vi "QT_DynCall.vi"(0 "QT Ref In":T11, 1 "Frame Grabber Settings":T15={"Name"="", "Digitizer"=0, "Input"=0, "Width"=0, "Height"=0, "Input format"=enum."PAL", "Frame rate"=0.0, "Reserved"=0, "Dialogs"=0} {"Frame rate" format="%#1_6g"; "Dialogs" format="%.0b"}, 3 "Compression Settings":T14 {"Dialogs" format="%.0b"; "Comp. Quality" format="%.0x"; "Codec" format="%.0x"}, 4 "Movie Settings":T10 {"Dialogs" format="%.0b"}, 5 "Image in":T5 {"Dialogs" format="%.0b"}, 6 "Sound in":T4 {"Rate" format="%x"}, 7 "error in (no error)":errorcluster, 8 "Selector":T16=enum."Get QT & CIN info", 9 "Video Settings in":T3={"Color format"=1, "Hue"=0.0, "Saturation"=0.0, "Brightness"=0.0, "Contrast"=0.0, "Sharpness"=0.0, "Black Level"=0.0, "White Level"=0.0, "Options"=0, "Dialogs"=0} {"Dialogs" format="%.0b"; "Color format" items=["Black & White (8 bits)", "RGB (24 bits)", "RGBx (32 bits)", "RGBA (32bits)", "RGB B&W (32 bits)", "HSI (24 bits)", "HSIx (32 bits)", "HSI B&W (32 bits)"]; "Brightness" format="%.2f"; "Contrast" format="%.2f"; "Sharpness" format="%.2f"; "Black Level" format="%.2f"; "White Level" format="%.2f"; "Saturation" format="%.2f"; "Hue" format="%.2f"}, 12 "Private":T6={"reserved 1"=4, "reserved 2"=0, "reserved 3"=0, "reserved 4"=0}, 13 "Effect":T9 {"Matrix" format="%.2f"}, 15 "File Settings":T13 {"Dialogs" format="%.0b"}) -> (16 "Info Out":T12, 17 "Video Settings out":T3={"Color format"=1, "Hue"=0.0, "Saturation"=0.0, "Brightness"=0.0, "Contrast"=0.0, "Sharpness"=0.0, "Black Level"=0.0, "White Level"=0.0, "Options"=0, "Dialogs"=0} {"Dialogs" format="%.0b"; "Color format" items=["Black & White (8 bits)", "RGB (24 bits)", "RGBx (32 bits)", "RGBA (32bits)", "RGB B&W (32 bits)", "HSI (24 bits)", "HSIx (32 bits)", "HSI B&W (32 bits)"]; "Brightness" format="%.2f"; "Contrast" format="%.2f"; "Sharpness" format="%.2f"; "Black Level" format="%.2f"; "White Level" format="%.2f"; "Saturation" format="%.2f"; "Hue" format="%.2f"}, 20 "QT Ref Out":T11, 23 "Movie info":T7 {"Tracks"."Rate" format="%.2f"}, 24 "QT Info":T1 {"Digitizers"."In Flags" format="%.0b"; "Digitizers"."Out Flags" format="%.0b"; "Digitizers"."Inputs" items=["Composite", "S-Video", "RGB", "RGB Synch", "YUV", "YUV Synch", "TV Tuner", "sdiln"]; "CIN rev ID" format="%.2f"}, 25 "Image/Movie Out":T5 {"Dialogs" format="%.0b"}, 26 "Sound out":T4 {"Rate" format="%x"}, 27 "error out":errorcluster={"status"=TRUE, "code"=-43, "source"=""})   [LabVIEW 2024]
uses:
  <userlib>/ImageProcessing/QTLIB_2595_LV86/QT_Image.ctl
  <userlib>/ImageProcessing/QTLIB_2595_LV86/QT_Digitizer.ctl
  <userlib>/ImageProcessing/QTLIB_2595_LV86/QT_Info.ctl
  <userlib>/ImageProcessing/QTLIB_2595_LV86/QT_Selector.ctl
  <userlib>/ImageProcessing/QTLIB_2595_LV86/QT_Ref.ctl
  <userlib>/ImageProcessing/QTLIB_2595_LV86/QT_Sound.ctl
  <userlib>/ImageProcessing/QTLIB_2595_LV86/QT_Video.ctl
  <userlib>/ImageProcessing/QTLIB_2595_LV86/QT_ErrInfo.ctl
  <userlib>/ImageProcessing/QTLIB_2595_LV86/QT_Private.ctl
  <userlib>/ImageProcessing/QTLIB_2595_LV86/QT_Compression.ctl
  <userlib>/ImageProcessing/QTLIB_2595_LV86/QT_File.ctl
  <userlib>/ImageProcessing/QTLIB_2595_LV86/QT_FrameGrabber.ctl
  <userlib>/ImageProcessing/QTLIB_2595_LV86/QT_Track.ctl
  <userlib>/ImageProcessing/QTLIB_2595_LV86/QT_MovieInfo.ctl
  <userlib>/ImageProcessing/QTLIB_2595_LV86/QT_Movie.ctl
  <userlib>/ImageProcessing/QTLIB_2595_LV86/QT_Effect.ctl
panel:
  # "[0,0] [0,1]  [0,2] [1,0].. [2,2]"
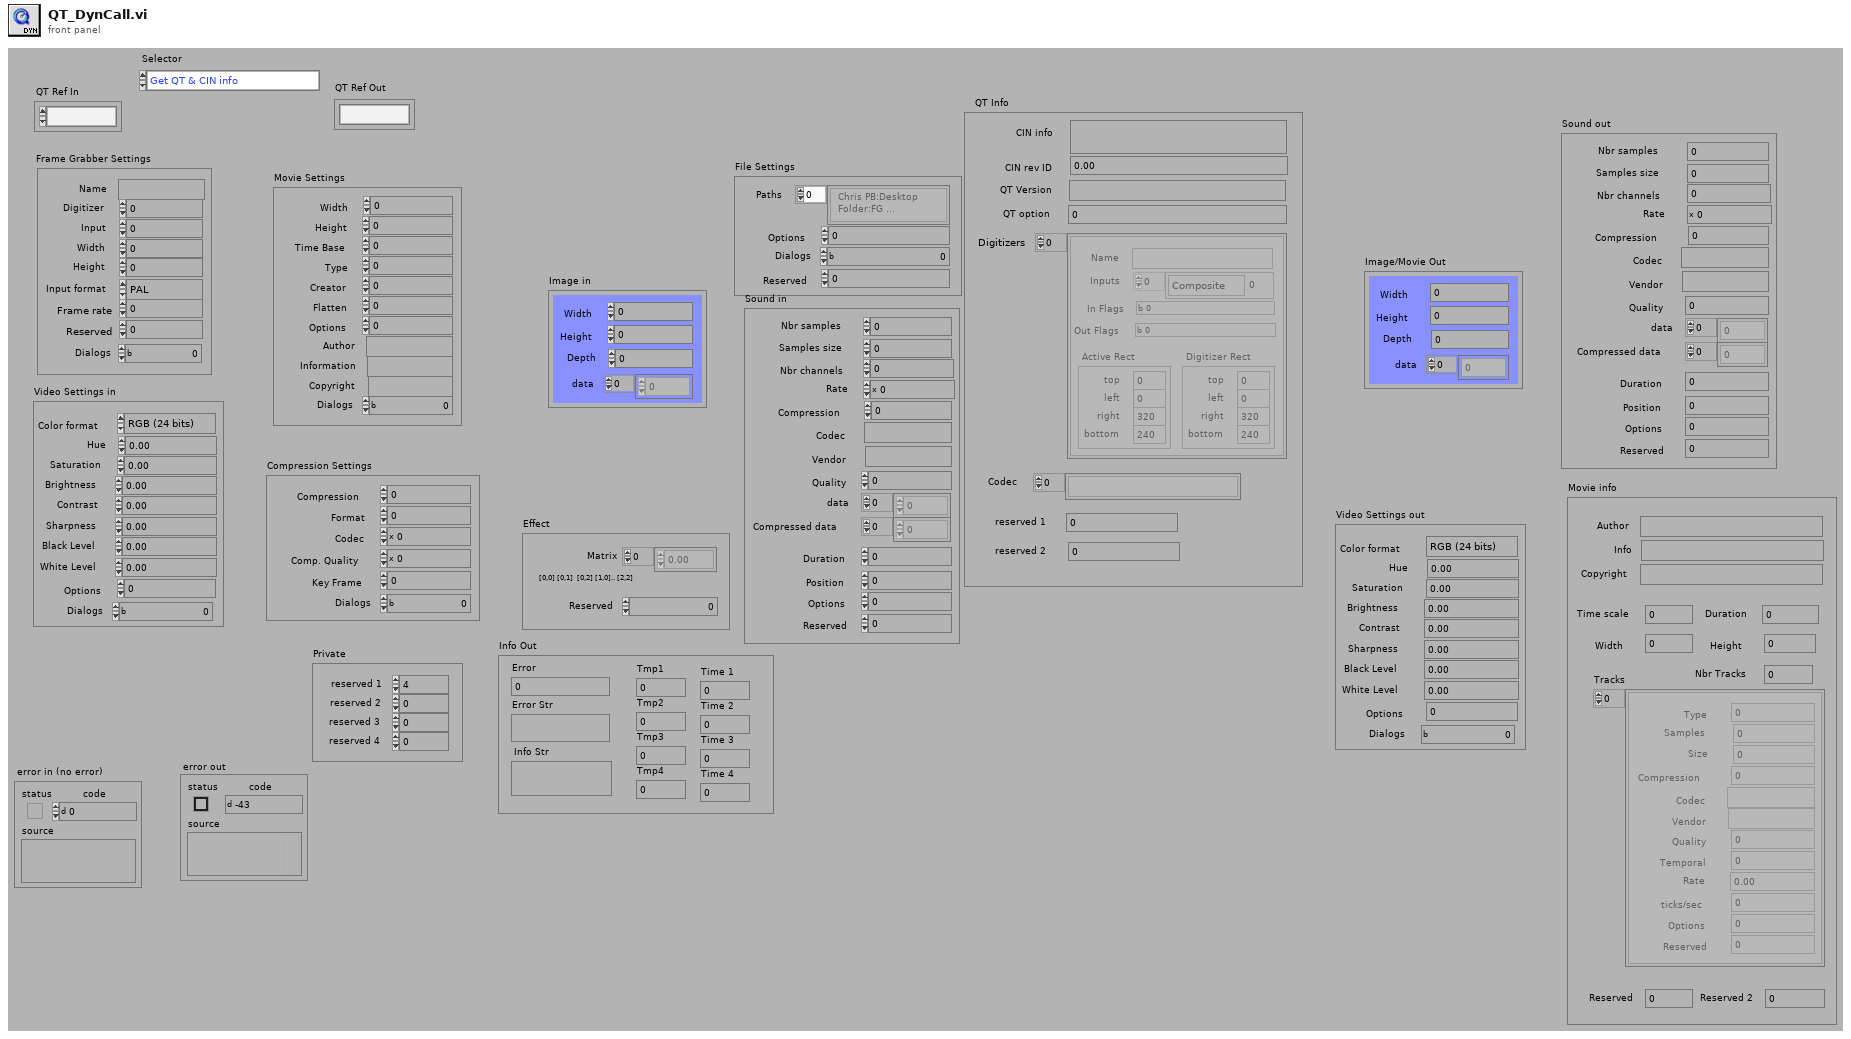
[diagram p1: front panel]
types:
  T1 = typedef "QT_Info.ctl" = cluster{"CIN info":string, "CIN rev ID":dbl, "QT Version":string, "QT option":i32, "Digitizers\n":T2[], "Codec":string[], "reserved 1":i32, "reserved 2":i32}
  T2 = typedef "QT_Digitizer.ctl" = cluster{"Name":string, "Inputs":i32[], "In Flags":i32, "Out Flags":i32, "Digitizer Rect":cluster{"top":i32, "left":i32, "right":i32, "bottom":i32}, "Active Rect":cluster{"top":i32, "left":i32, "right":i32, "bottom":i32}}
  T3 = typedef "QT_Video.ctl" = cluster{"Color format":u32, "Hue":dbl, "Saturation":dbl, "Brightness":dbl, "Contrast":dbl, "Sharpness":dbl, "Black Level":dbl, "White Level":dbl, "Options":i32, "Dialogs":u32}
  T4 = typedef "QT_Sound.ctl" = cluster{"Nbr samples":i32, "Samples size":i32, "Nbr channels":i32, "Rate ":i32, "Compression":i32, "Codec":string, "Vendor":string, "Quality":i32, "data":i16[], "Compressed data":u8[], "Duration":i32, "Position":i32, "Options":i32, "Reserved":i32}
  T5 = typedef "QT_Image.ctl" = cluster{"Width":i32, "Height":i32, "Depth":i32, "data":u8[], "Compressed data":u8[], "Color table":u32[], "Duration":i32, "Options":i32, "Timestamp":i32, "ID":i32, "Reserved":i32, "Dialogs":u32}
  T6 = typedef "QT_Private.ctl" = cluster{"reserved 1":i32, "reserved 2":i32, "reserved 3":i32, "reserved 4":i32}
  T7 = typedef "QT_MovieInfo.ctl" = cluster{"Author":string, "Info":string, "Copyright":string, "Time scale":i32, "Duration":i32, "Width":i32, "Height":i32, "Nbr Tracks":i32, "Tracks":T8[], "Reserved":i32, "Reserved 2":i32}
  T8 = typedef "QT_Track.ctl" = cluster{"Type":i32, "Samples":i32, "Size":i32, "Compression":i32, "Codec":string, "Vendor":string, "Quality":i32, "Temporal":i32, "Rate ":dbl, "ticks/sec":i32, "Options":i32, "Reserved":i32}
  T9 = typedef "QT_Effect.ctl" = cluster{"Reserved":i32, "Matrix":dbl[]}
  T10 = typedef "QT_Movie.ctl" = cluster{"Width":i32, "Height":i32, "Time Base":i32, "Type":i32, "Creator":i32, "Flatten":i32, "Options":i32, "Author":string, "Information":string, "Copyright":string, "Dialogs":u32}
  T11 = typedef "QT_Ref.ctl" = refnum<k1>
  T12 = typedef "QT_ErrInfo.ctl" = cluster{"Error":i32, "Error Str":string, "Info Str":string, "Tmp1":i32, "Tmp2":i32, "Tmp3":i32, "Tmp4":i32, "Time 1":i32, "Time 2":i32, "Time 3":i32, "Time 4":i32}
  T13 = typedef "QT_File.ctl" = cluster{"Paths":string[], "Options":i32, "Dialogs":u32, "Reserved":i32}
  T14 = typedef "QT_Compression.ctl" = cluster{"Compression":i32, "Format":i32, "Codec":i32, "Comp. Quality":i32, "Key Frame":i32, "Dialogs":u32}
  T15 = typedef "QT_FrameGrabber.ctl" = cluster{"Name":string, "Digitizer":i32, "Input":i32, "Width":i32, "Height":i32, "Input format":enum32{"NTSC", "PAL", "Secam"}, "Frame rate":dbl, "Reserved":i32, "Dialogs":u32}
  T16 = typedef "QT_Selector.ctl" = enum32{"do nothing", "Get all Sources", "Get Source info", "Open Image", "Save Image to File", "Effect", "Close", "SG Grab", "Compress in Memory", "Decompress to Memory", "New Movie", "Open Movie", "Add Frame", "Get Frame", "Close Movie", "Get QT & CIN info", "SG init", "SG Close", "Open sound file", "Close sound file", "Read sound data", "Write sound data", "Import sound", "Export sound", "Add sound to movie", "Get sound from movie", "reserved", "reserved 1", "reserved 2"}
  T17 = enum32{"invalid CPU target", "Motorola 68K", "PowerPC", "Intel x86", "SPARC", "PA-RISC", "MIPS", "Alpha"}
  T18 = enum32{"invalid OS target", "Mac OS", "Windows 3.1", "Windows 95/NT", "Solaris 1", "Solaris 2", "HP-UX", "PowerMAX", "Linux", "Irix", "Rhapsody", "BeOS", "AIX", "OSF1", "VxWorks", "PharLap", "Carbon", "RTX", "Windows x64", "Linux x64", "Mac OS X x64"}
  T19 = enum32{"invalid CPU target", "Motorola 68K", "PowerPC", "Intel x86", "SPARC", "PA-RISC", "MIPS", "Alpha", "ARM", "AMD/Intel x64", "ARM64"}
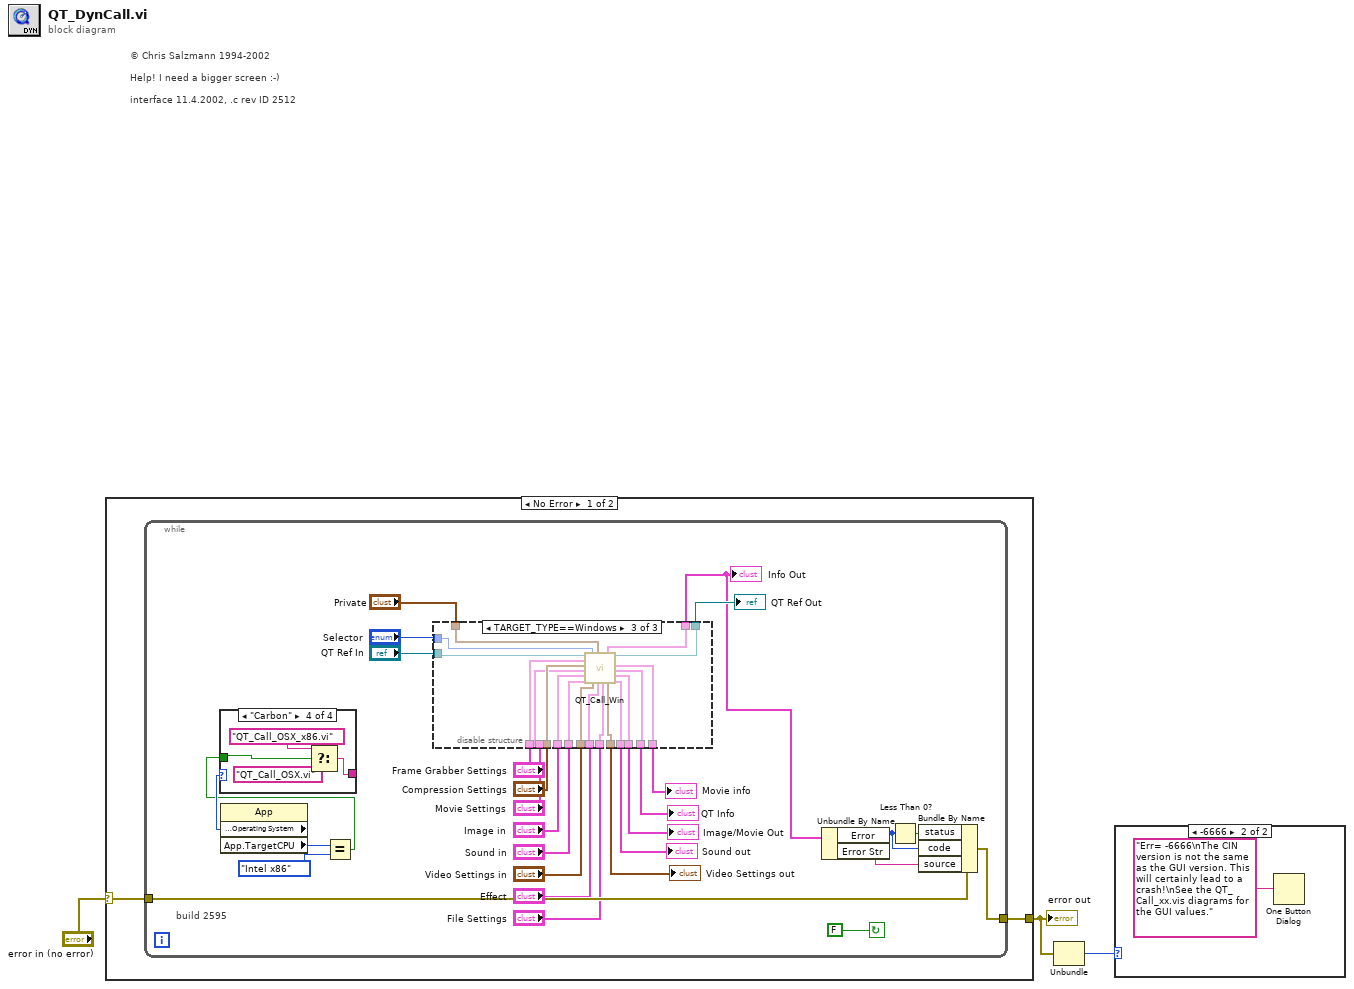
[diagram p0: block diagram]
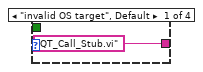
[diagram p3: hidden frame]
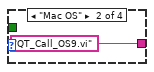
[diagram p4: hidden frame]
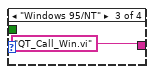
[diagram p5: hidden frame]
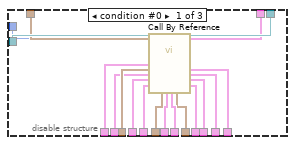
[diagram p6: hidden frame]
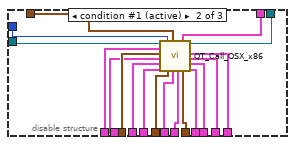
[diagram p7: hidden frame]
diagram:
  # "© Chris Salzmann 1994-2002\n\nHelp! I need a bigger screen :-)\n\ninterface 11.4.2002, .c rev ID 2512"
  n1 = case shown="No Error" "error in (no error)" {
    selector: "error in (no error)" -> [w4 w99]
    tunnel: [w5 w99] -> w2
    frame No Error {
      n2 = while {
        tunnel: [w13] -> w5
        tunnel: w4 -> [w33]
        stop <- FALSE continue-if-true
        # "build 2595"
        n3 = property class="App"() -> ("Application:Target:Operating System"=w12:T18, "App.TargetCPU"=w11:T19)  [unwired: 2 in, 2 out]
        n4 = Equal?(x=w11, y=T17."Intel x86") -> (x = y?=w9:bool)
        n5 = case shown="\"Carbon\"" w12 {
          tunnel: ["QT_Call_Stub.vi" ("name or relative path") "QT_Call_OS9.vi" ("name or relative path") "QT_Call_Win.vi" ("name or relative path") w38] -> _
          tunnel: w9 -> [_ _ _ w37]
          frame "invalid OS target", Default {
          }
          frame "Mac OS" {
          }
          frame "Windows 95/NT" {
          }
          frame "Carbon" {
            n6 = Select(t="QT_Call_OSX_x86.vi" ("name or relative path"), s=w37, f="QT_Call_OSX.vi" ("name or relative path")) -> (s? t:f=w38:string)
          }
        }
        n7 = disable-structure shown="TARGET_TYPE==Windows" {
          disable-tunnel: "QT Ref In" -> [w60 w80 w98]
          disable-tunnel: [w59 w76 w94] -> w30
          disable-tunnel: [w58 w77 w95] -> w29
          disable-tunnel: "Private" -> [w57 w78 w96]
          disable-tunnel: "Frame Grabber Settings" -> [w56 w75 w93]
          disable-tunnel: "Compression Settings" -> [w55 w74 w92]
          disable-tunnel: "Movie Settings" -> [w54 w73 w91]
          disable-tunnel: "Image in" -> [w53 w72 w90]
          disable-tunnel: "Sound in" -> [w52 w71 w89]
          disable-tunnel: "Video Settings in" -> [w51 w70 w88]
          disable-tunnel: "Effect" -> [w50 w69 w87]
          disable-tunnel: "File Settings" -> [w49 w68 w86]
          disable-tunnel: [w48 w67 w85] -> w19
          disable-tunnel: [w47 w63 w81] -> w18
          disable-tunnel: [w46 w66 w84] -> w17
          disable-tunnel: [w45 w65 w83] -> w16
          disable-tunnel: "Selector" -> [w44 w79 w97]
          disable-tunnel: [w43 w64 w82] -> w14
          frame condition #0 {
            n8 = call-by-ref "?"("QT Ref In"=w60, "Frame Grabber Settings"=w56, "Compression Settings"=w55, "Movie Settings"=w54, "Image in"=w53, "Sound in"=w52, "Selector"=w44, "Video Settings in"=w51, "Private"=w57, "Effect"=w50, "File Settings"=w49) -> (reference=w41:refnum<vi>, reference out=w61:refnum<vi>, error in=w62:errorcluster, error out=w42:errorcluster, "Info Out"=w58:T12, "Video Settings out"=w48:T3, "QT Ref Out"=w59:T11, "Movie info"=w47:T7, "QT Info"=w43:T1, "Image/Movie Out"=w45:T5, "Sound out"=w46:T4)  [unwired: 2 in]
          }
          frame condition #1 (active) {
            n9 = call <userlib>:"QT_Call_OSX_x86.vi"("QT Ref In"=w80, "Frame Grabber Settings"=w75, "Compression Settings"=w74, "Movie Settings"=w73, "Image in"=w72, "Sound in"=w71, "Selector"=w79, "Video Settings in"=w70, "Private"=w78, "Effect"=w69, "File Settings"=w68) -> ("Info Out"=w77:T12, "Video Settings out"=w67:T3, "QT Ref Out"=w76:T11, "Movie info"=w63:T7, "QT Info"=w64:T1, "Image/Movie Out"=w65:T5, "Sound out"=w66:T4)  [unwired: 2 in]
          }
          frame condition #2 {
            n10 = call <userlib>:"QT_Call_Win.vi"("QT Ref In"=w98, "Frame Grabber Settings"=w93, "Compression Settings"=w92, "Movie Settings"=w91, "Image in"=w90, "Sound in"=w89, "Selector"=w97, "Video Settings in"=w88, "Private"=w96, "Effect"=w87, "File Settings"=w86) -> ("Info Out"=w95:T12, "Video Settings out"=w85:T3, "QT Ref Out"=w94:T11, "Movie info"=w81:T7, "QT Info"=w82:T1, "Image/Movie Out"=w83:T5, "Sound out"=w84:T4)  [unwired: 2 in]
          }
        }
        "Video Settings out" <- w19
        "Sound out" <- w17
        "Image/Movie Out" <- w16
        "Movie info" <- w18
        "QT Ref Out" <- w30
        "Info Out" <- w29
        "QT Info" <- w14
        n11 = Unbundle By Name(w29) -> ("Error"=w7:i32, "Error Str"=w6:string)
        n12 = Less Than 0?(x=w7) -> (x < 0?=w8:bool)
        n13 = Bundle By Name(cluster=w33, "status"=w8, "code"=w7, "source"=w6) -> (w13:errorcluster)
      }
    }
    frame Error {
    }
  }
  "error out" <- w2
  n14 = Unbundle(w2) -> ("code"=w1:i32)  [unwired: 2 out]
  n15 = case shown="-6666" w1 {
    frame 0, Default {
    }
    frame -6666 {
      n16 = One Button Dialog(message="Err= -6666\nThe CIN version is not the same as the GUI version. This will certainly lead to a crash!\nSee the QT_Call_xx.vis diagrams for the GUI values.") -> ()  [unwired: 2 out]
    }
  }
